vi "Obtain Model.vi"(0 "Serial port asssistant model in":refnum<class "Serial port assistant model.lvclass">, 7 "init information":string, 11 "error in (no error)":errorcluster) -> (4 "Serial port asssistant model out":refnum<class "Serial port assistant model.lvclass">, 15 "error out":errorcluster)   [LabVIEW 2022 SP3, in "Serial port assistant model.lvlib" / "Serial port assistant model.lvclass"]
uses:
  Serial port assistant model.lvclass
  changed data--type.ctl
  Serial port assistant model.lvclass/Serial port assistant model.ctl
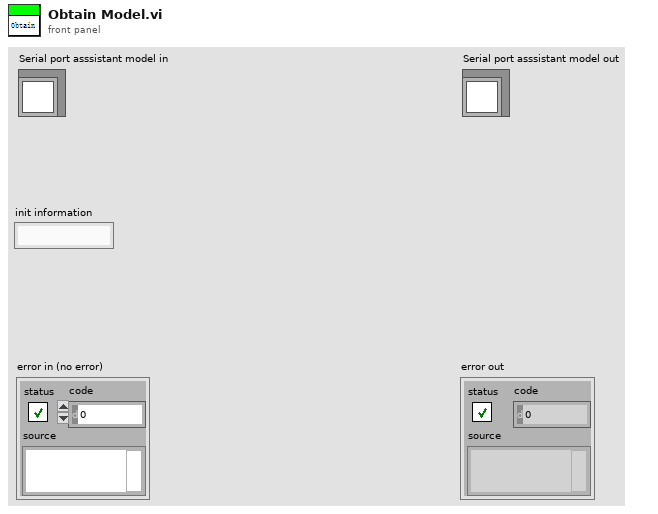
[diagram p1: front panel]
types:
  T1 = typedef "Serial port assistant model.lvlib/Serial port assistant model.lvclass/changed data--type.ctl" = cluster{"changed data":string}
  T2 = typedef "Rendezvous RefNum" = refnum<k1>
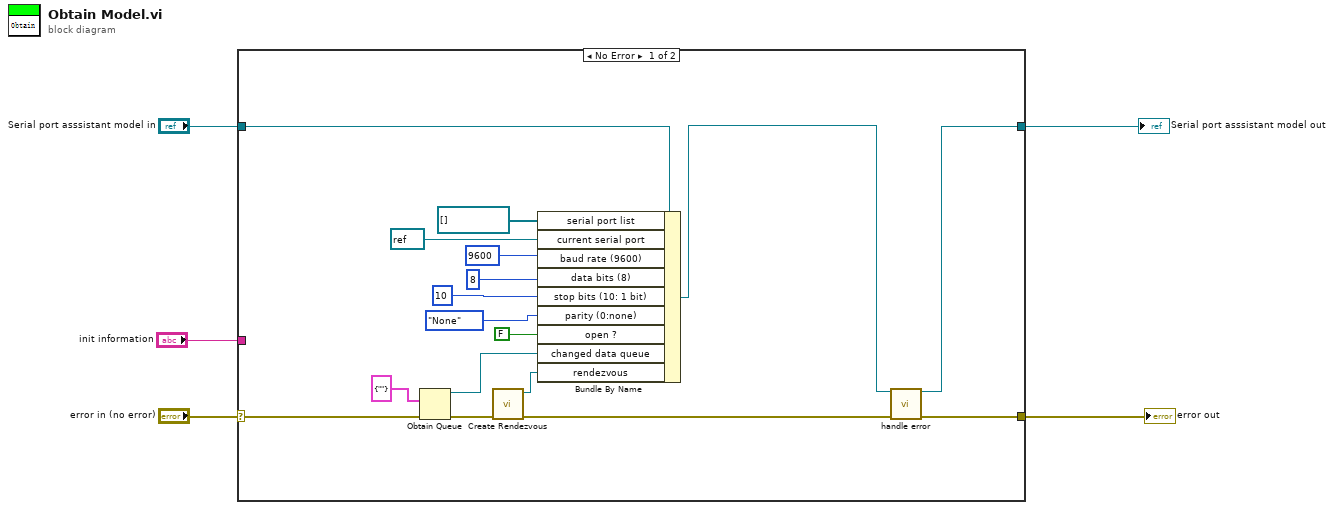
[diagram p0: block diagram]
diagram:
  n1 = case shown="No Error" "error in (no error)" {
    selector: "error in (no error)" -> [w14 w24]
    tunnel: [w8 w24] -> w4
    tunnel: "Serial port asssistant model in" -> [w22 w23]
    tunnel: [w6 w23] -> w2
    tunnel: "init information" -> [_ _]
    frame No Error {
      n2 = Obtain Queue(element data type=T1 {"changed data"=""} ("changed data"), error in (no error)=w14) -> (queue out=w12:refnum<queue>, error out=w11:errorcluster)  [unwired: 3 in, 1 out]
      n3 = call <vilib>:"Create Rendezvous.vi"("error in (no error)"=w11) -> ("error out"=w9:errorcluster, "rendezvous"=w10:T2)  [unwired: 4 in, 1 out]
      n4 = Bundle By Name(cluster=w22, "serial port list"=refnum<visa-resource-name>[] [], "current serial port"=refnum<visa-resource-name> refnum, "baud rate (9600)"=u32 9600, "data bits (8)"=u16 8, "stop bits (10: 1 bit)"=u16 10, "parity (0:none)"=enum16{"None", "Odd", "Even", "Mark", "Space"}."None", "open ?"=FALSE, "changed data queue"=w12, "rendezvous"=w10) -> (w7:refnum<class "Serial port assistant model.lvclass">)
      n5 = call "handle error.vi"("Serial port assistant model in"=w7, "error in (no error)"=w9) -> ("Serial port assistant model out"=w6:refnum<class "Serial port assistant model.lvclass">, "error out"=w8:errorcluster)  [unwired: 12 in]
    }
    frame Error {
    }
  }
  "error out" <- w4
  "Serial port asssistant model out" <- w2
